vi "Engine - Error - Runtime.vi"(8 "error in (no error)":errorcluster, 9 "Iteration":u32, 10 "Runtime Status Channels In":dbl[](array[numeric])) -> (0 "error out":errorcluster, 2 "Runtime Status Channels In":dbl[](array[numeric]))   [LabVIEW 2015, in "DMM-SWITCH-ScanList Engine.lvlib"]
doc: "Add Runtime Status and Error Information to Output Channels dedicated for Runtime Status."
uses:
  DMM-SWITCH-ScanList Engine.lvlib
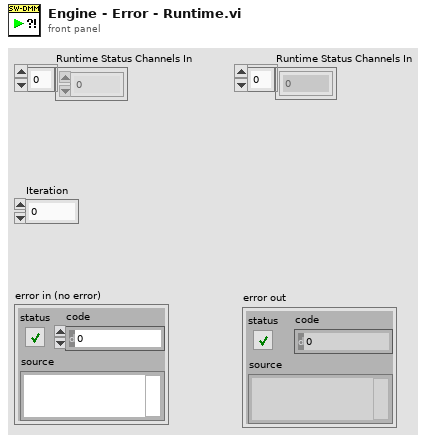
[diagram p1: front panel]
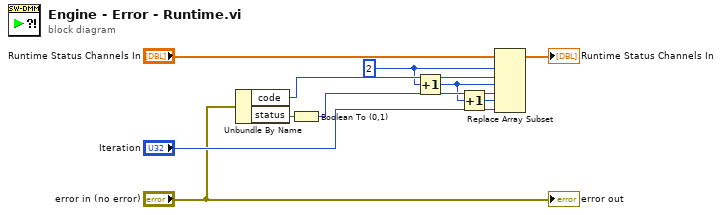
[diagram p0: block diagram]
diagram:
  w3 = 2 ("index")
  n1 = Unbundle By Name("error in (no error)") -> ("code"=w4:i32, "status"=w7:bool)
  n2 = Boolean To (0,1)(Boolean=w7) -> (0, 1=w5:i16)
  n3 = Increment(x=w3) -> (x+1=w1:i32)
  n4 = Increment(x=w1) -> (x+1=w2:i32)
  n5 = Replace Array Subset(array="Runtime Status Channels In", new element #1=w4, index #1=w3, new element #2=w5, index #2=w1, new element #3="Iteration", index #3=w2) -> (→"Runtime Status Channels In":dbl[])
  "error out" <- "error in (no error)"
